vi "QueryServer_SetResponse_Invoke.vi"(0 "gRPCid":T1, 2 "status":i32, 3 "error in (no error)":errorcluster) -> (10 "error out":errorcluster)   [LabVIEW 2019, in "labview-grpc-query-server.lvlib"]
uses:
  labview-grpc-query-server.lvlib
  QueryServer_gRPCid.ctl
  QueryServer_InvokeResponse.ctl
  build/Debug/labview_grpc_server.dll
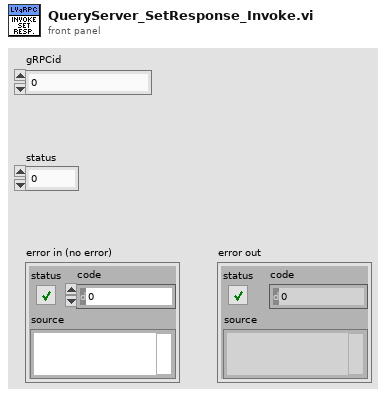
[diagram p1: front panel]
types:
  T1 = typedef "labview-grpc-query-server.lvlib/QueryServer_gRPCid.ctl" = u64
  T2 = typedef "labview-grpc-query-server.lvlib/QueryServer_InvokeResponse.ctl" = cluster{"status":i32}
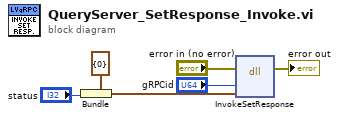
[diagram p0: block diagram]
diagram:
  n1 = Bundle(cluster=T2 {"status"=0} ("InvokeResponse"), "status"="status") -> (w3:T2)
  n2 = dll-call lib="C:/dev/labview-grpc-server/build/Debug/labview_grpc_server.dll" fn="InvokeSetResponse"(error in="error in (no error)", "id"="gRPCid", "data"=w3) -> (error out=→"error out":errorcluster)  [unwired: 5 in, 1 out]
